vi "ErrorLogFile_Init.vi"(0 "object in":refnum<class "ErrorLogFile.lvclass">, 2 "Folder":path, 5 "Error In":errorcluster, 8 "History":i32=30) -> (14 "object out":refnum<class "ErrorLogFile.lvclass">, 19 "Error Out":errorcluster)   [LabVIEW 2019, in "ErrorLogFile.lvclass"]
uses:
  ErrorLogFile.lvclass
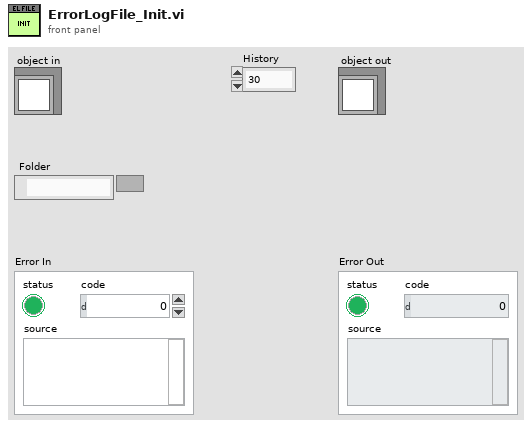
[diagram p1: front panel]
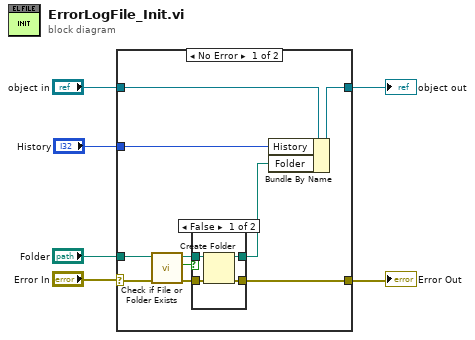
[diagram p0: block diagram]
diagram:
  n1 = case shown="No Error" "Error In" {
    selector: "Error In" -> [w11 w23]
    tunnel: "object in" -> [w16 w24]
    tunnel: [w15 w24] -> w5
    tunnel: [w10 w23] -> w3
    tunnel: "Folder" -> [w8 _]
    tunnel: "History" -> [w14 _]
    frame No Error {
      n2 = call <vilib>:"Check if File or Folder Exists.vi"("error in (no error)"=w11, "path"=w8) -> ("error out"=w12:errorcluster, "file or folder exists?"=w7:bool, "dup path"=w13:path)  [unwired: 7 in]
      n3 = case shown="False" w7 {
        tunnel: w13 -> [w20 w22]
        tunnel: w12 -> [w19 w21]
        tunnel: [w18 w21] -> w10
        tunnel: [w17 w22] -> w9
        frame False {
          n4 = Create Folder(path (use dialog)=w20, error in=w19) -> (created path=w17:path, error out=w18:errorcluster)  [unwired: 1 in, 1 out]
        }
        frame True {
        }
      }
      n5 = Bundle By Name(cluster=w16, "History"=w14, "Folder"=w9) -> (w15:refnum<class "ErrorLogFile.lvclass">)
    }
    frame Error {
    }
  }
  "object out" <- w5
  "Error Out" <- w3
